vi "nbp.vi"() -> ()   [LabVIEW 2026]
uses:
  <vilib>/httpClient/LabVIEWHTTPClient.lvlib
panel:
  out "Waveform Graph":dbl[](graph)
  out "concatenated string":string
  in  "Pobierz dane":bool
  in  "Data do":timestamp
  in  "Data od":timestamp
  in  "Enum":enum16{"USD", "EUR", "CHF"}(ring)
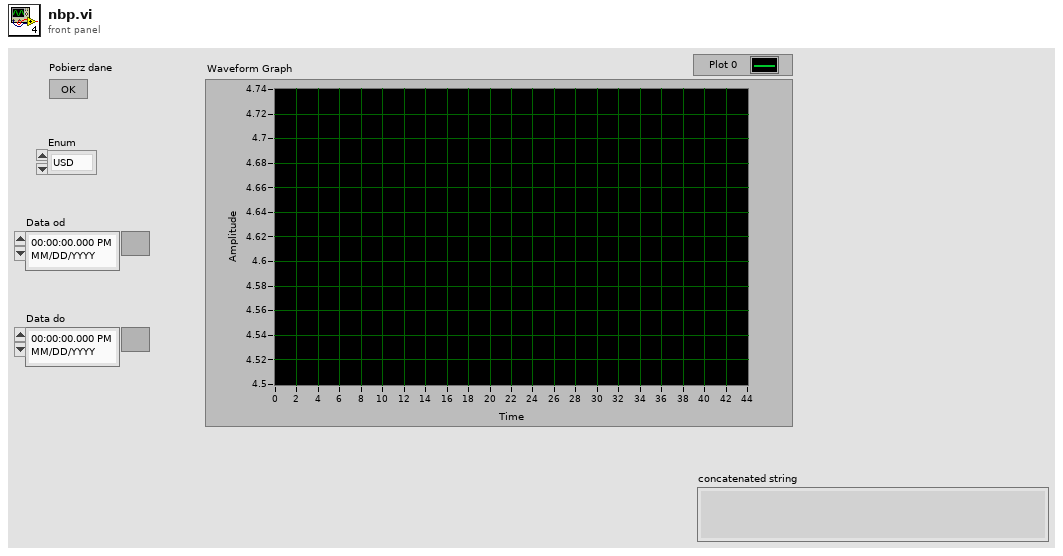
[diagram p1: front panel]
types:
  T1 = cluster{"table":string, "currency":string, "code":string, "rates":cluster{"no":string, "effectiveDate":string, "mid":dbl}[]}
  T2 = typedef "LabVIEWHTTPClient.lvlib/ClientHandle.ctl" = refnum<k1>
  T3 = cluster{"no":string, "effectiveDate":string, "mid":dbl}[]
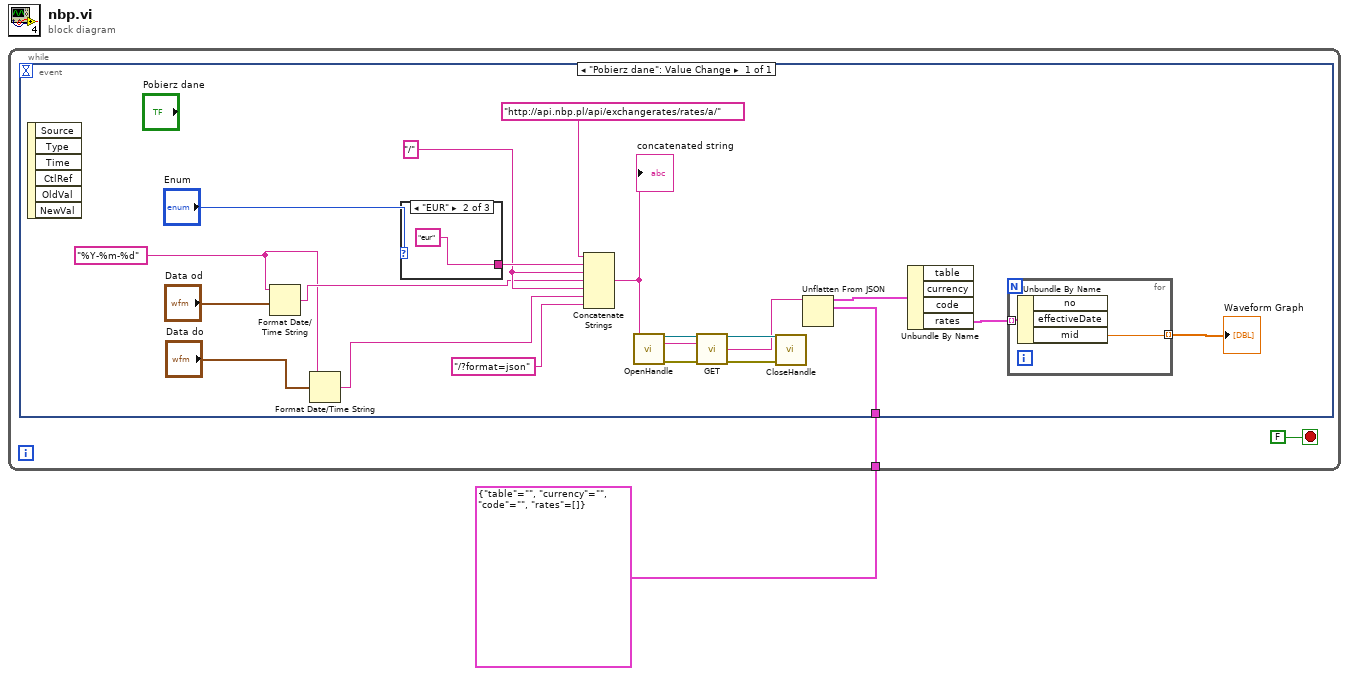
[diagram p0: block diagram]
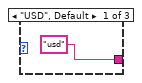
[diagram p2: hidden frame]
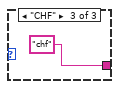
[diagram p3: hidden frame]
diagram:
  n1 = while {
    tunnel: T1 {"table"="", "currency"="", "code"="", "rates"=[]} -> [w2]
    stop <- FALSE stop-if-true
    n2 = event shown="[0] \"Pobierz dane\": Value Change" {
      selector: _ -> [_]
      dyn-events: _ -> [_]
      timeout: _ -> [_]
      tunnel: w2 -> [w8]
      event "Pobierz dane": Value Change {
        w20 = "/"
        w4 = "%Y-%m-%d"
        n3 = event-data() -> ()  [unwired: 1 in, 6 out]
        n4 = Format Date/Time String(time format string (%c)=w4, seconds (now)="Data od") -> (date/time string=w15:string)  [unwired: 1 in]
        n5 = Format Date/Time String(time format string (%c)=w4, seconds (now)="Data do") -> (date/time string=w16:string)  [unwired: 1 in]
        n6 = case shown="\"EUR\"" "Enum" {
          tunnel: ["usd" "eur" "chf"] -> w21
          frame "USD", Default {
          }
          frame "EUR" {
          }
          frame "CHF" {
          }
        }
        n7 = Concatenate Strings("http://api.nbp.pl/api/exchangerates/rates/a/", w21, w20, w15, w20, w16, "/?format=json") -> (w10:string)
        "concatenated string" <- w10
        n8 = call <vilib>:"OpenHandle.vi"() -> ("client handle out"=w14:T2, "error out"=w13:errorcluster)  [unwired: 14 in]
        n9 = call <vilib>:"GET.vi"("client handle"=w14, "url"=w10, "error in (no error)"=w13) -> ("client handle out"=w12:T2, "body"=w9:string, "error out"=w11:errorcluster)  [unwired: 9 in, 1 out]
        n10 = call <vilib>:"CloseHandle.vi"("client handle"=w12, "error in (no error)"=w11) -> ()  [unwired: 13 in, 1 out]
        n11 = Unflatten From JSON(JSON string=w9, type and defaults=w8) -> (value=w7:T1)  [unwired: 5 in, 1 out]
        n12 = Unbundle By Name(w7) -> ("rates"=w6:T3)  [unwired: 3 out]
        n13 = for {
          tunnel: w6 -> [w25] mode=indexing
          tunnel: [w24] -> w5 mode=indexing
          n14 = Unbundle By Name(w25) -> ("mid"=w24:dbl)  [unwired: 2 out]
        }
        "Waveform Graph" <- w5
      }
    }
  }
